vi "GOOP_LVClass_Global_OnCommand.vi"(10 "Command ID":string, 11 "Object":u64) -> ()   [LabVIEW 2020]
doc: "NI Confidential \n\n/**\n@brief This VI is called by the framework when the user selects a menu item on this item in the tree.\n\n@author Joel Dixon\n\n@par Sample_Item_OnCommand.vi\n The VI should contain a switch statement on the CommandID parameter to select the appropriate command and take the desired action for the command. See the description of the CommandID parameter for more information. \n\n@param \"Command ID\" [in] \nThe tag of the command to be performed. Corresponds to the Menu Tag field in the Menu Items cluster passed to mxLvSetPopupMenu.vi.\n*/"
uses:
  <resource>/Framework/Providers/Open_GDS/ClassProviders/Provider_BaseClassInterface/ClassWriter_class/ClassWriter.lvclass
  <resource>/Framework/Providers/Open_GDS/SubVIs/GOOP_UMLEditor_CallMainAction.ctl
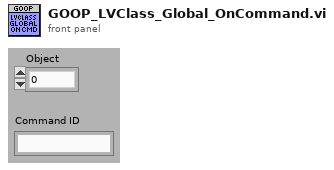
[diagram p1: front panel]
types:
  T1 = enum32{"None", "Stop", "Question", "Exclamation", "Information"}
  T2 = typedef "GOOP_UMLEditor_CallMainAction.ctl" = enum16{"OpenUmlEditor", "ReverseEngineering:WholeProject", "ReverseEngineering:OneClass", "ReverseEngineering:OneVI", "ShowInStateDiagram:OneVI", "OpenUMLFile"}
  T3 = enum32{"Bad", "Idle", "Run top level", "Running"}
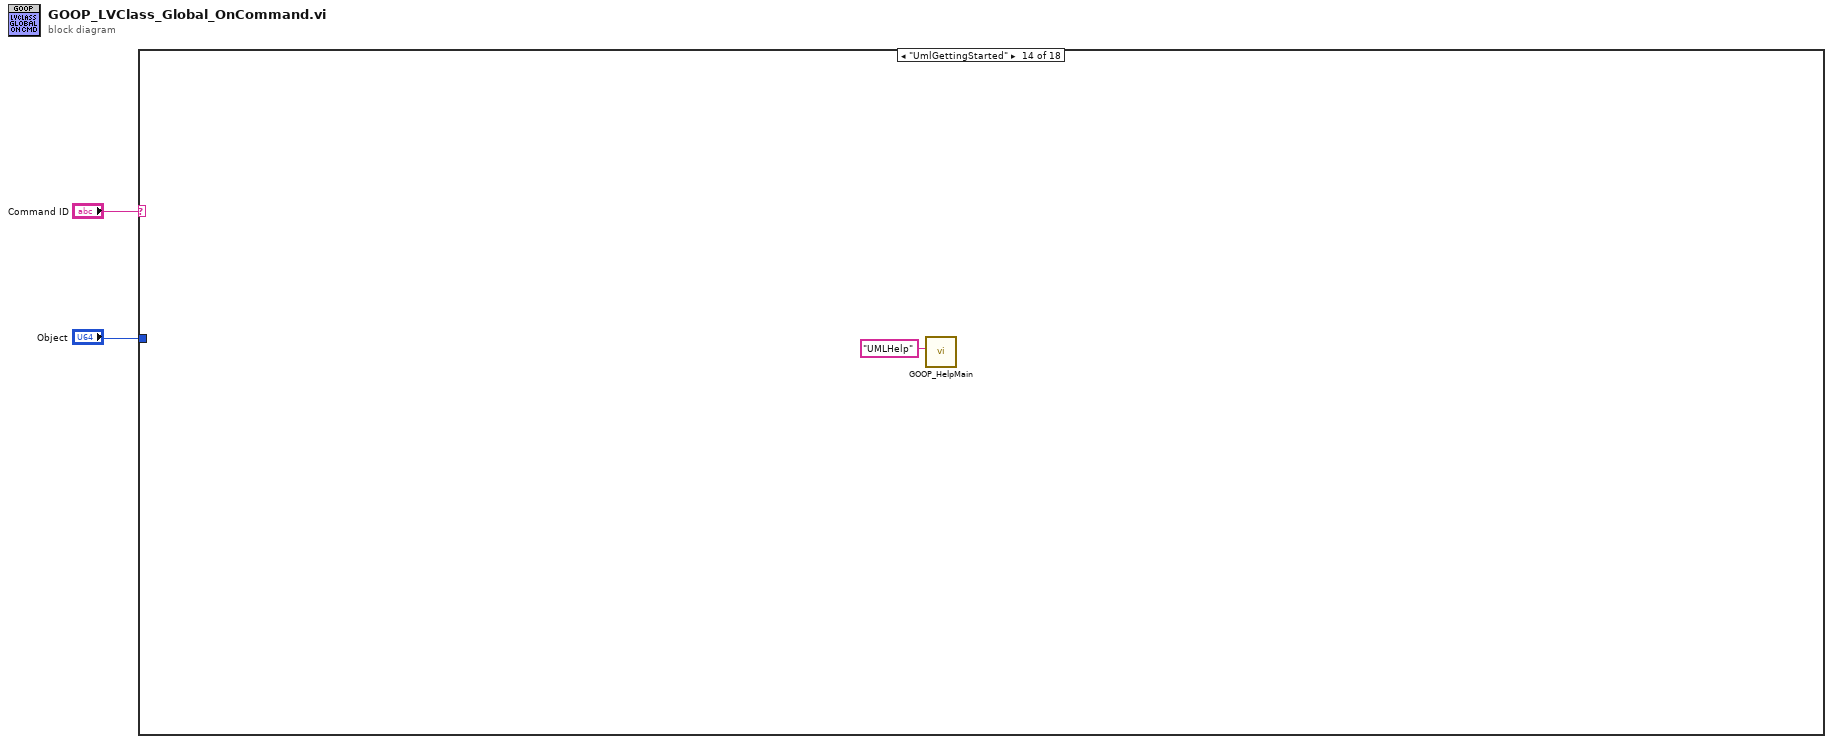
[diagram p0: block diagram]
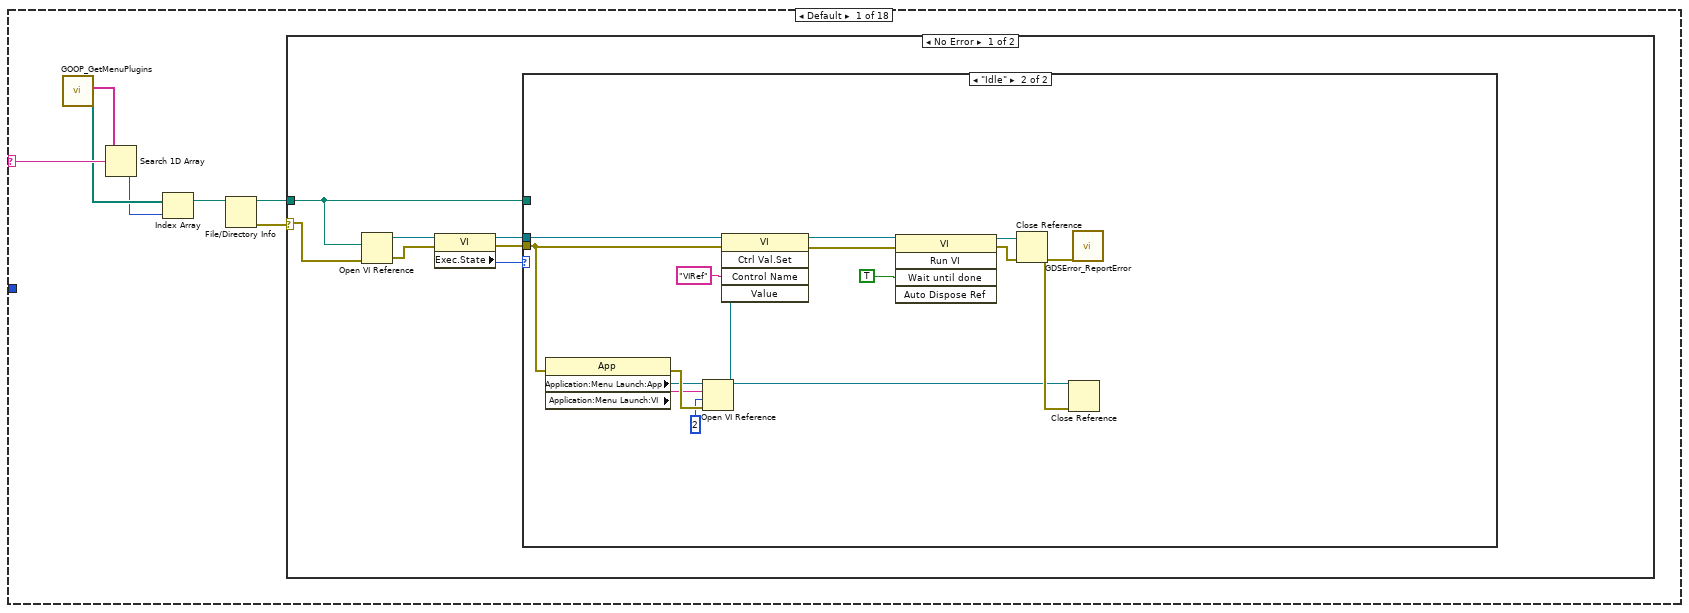
[diagram p2: hidden frame]
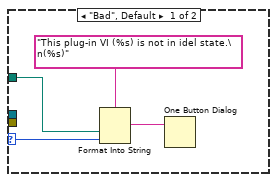
[diagram p3: hidden frame]
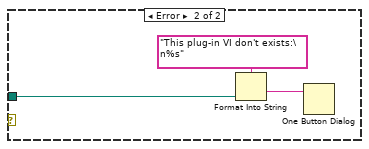
[diagram p4: hidden frame]
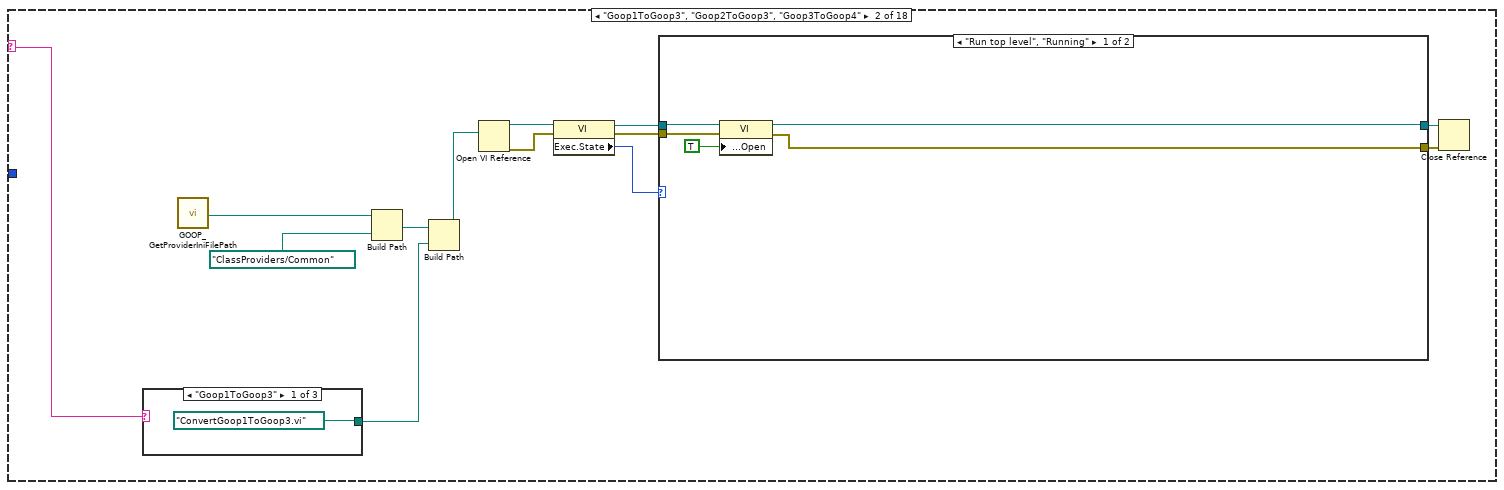
[diagram p5: hidden frame]
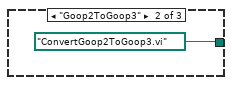
[diagram p6: hidden frame]
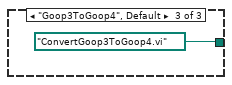
[diagram p7: hidden frame]
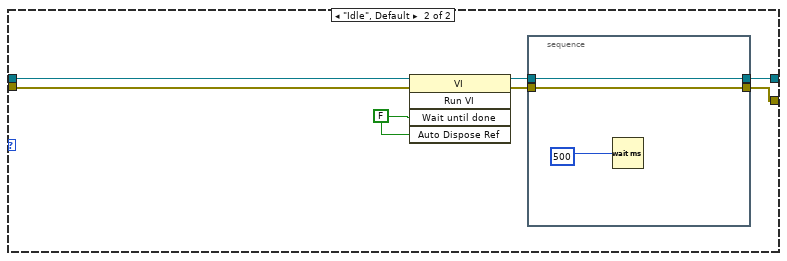
[diagram p8: hidden frame]
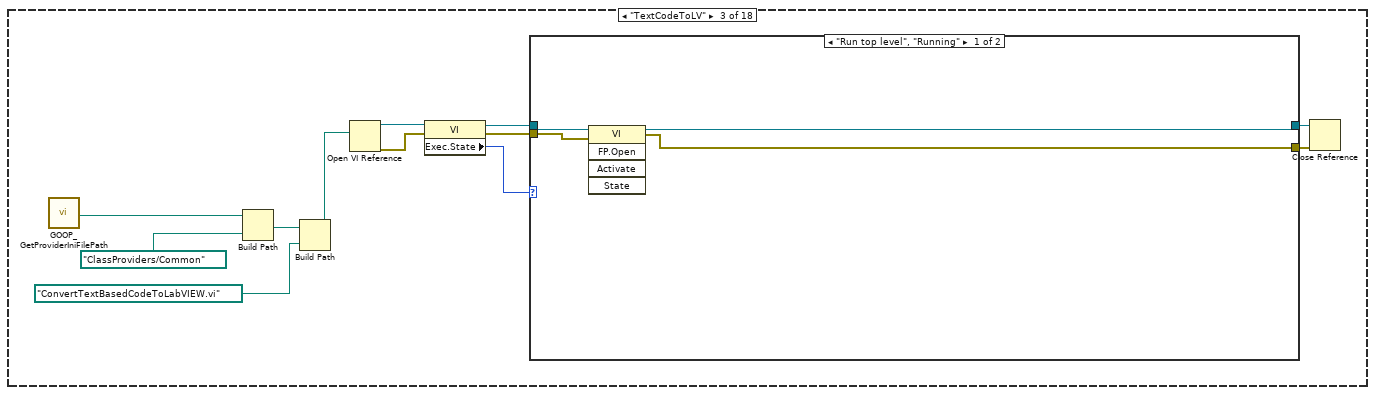
[diagram p9: hidden frame]
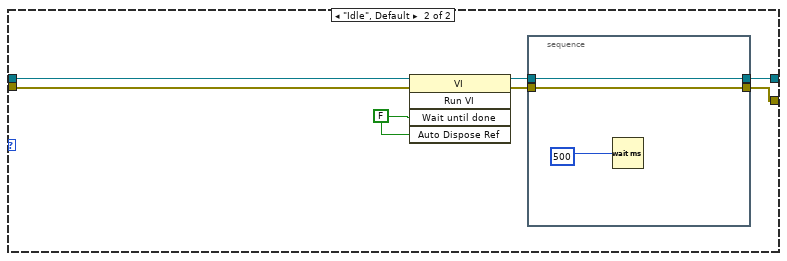
[diagram p10: hidden frame]
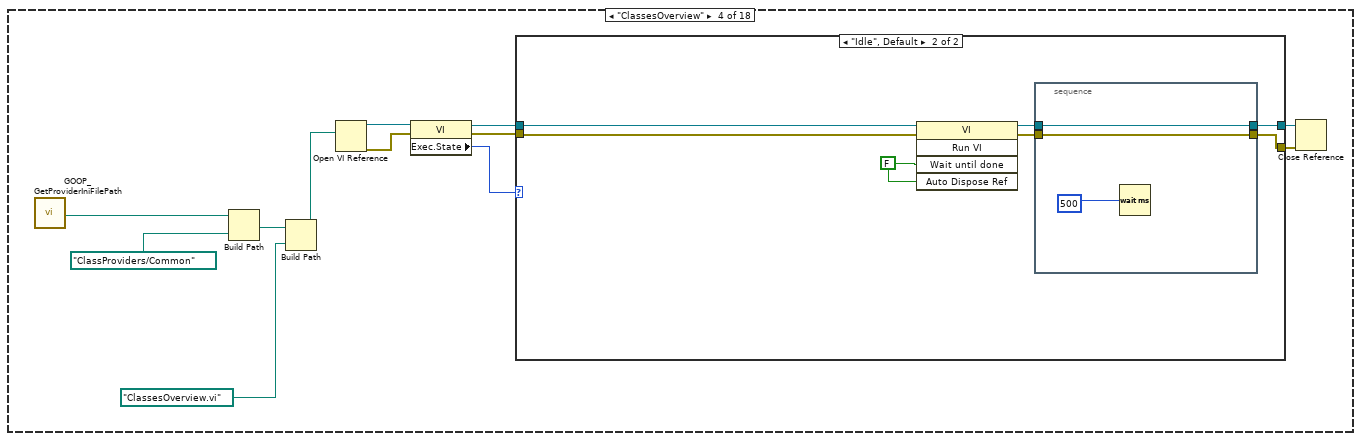
[diagram p11: hidden frame]
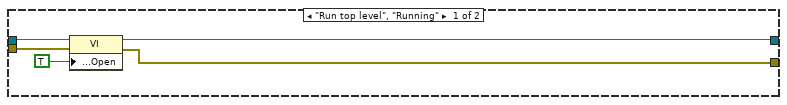
[diagram p12: hidden frame]
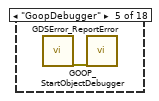
[diagram p13: hidden frame]
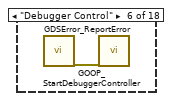
[diagram p14: hidden frame]
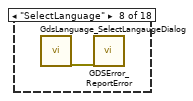
[diagram p16: hidden frame]
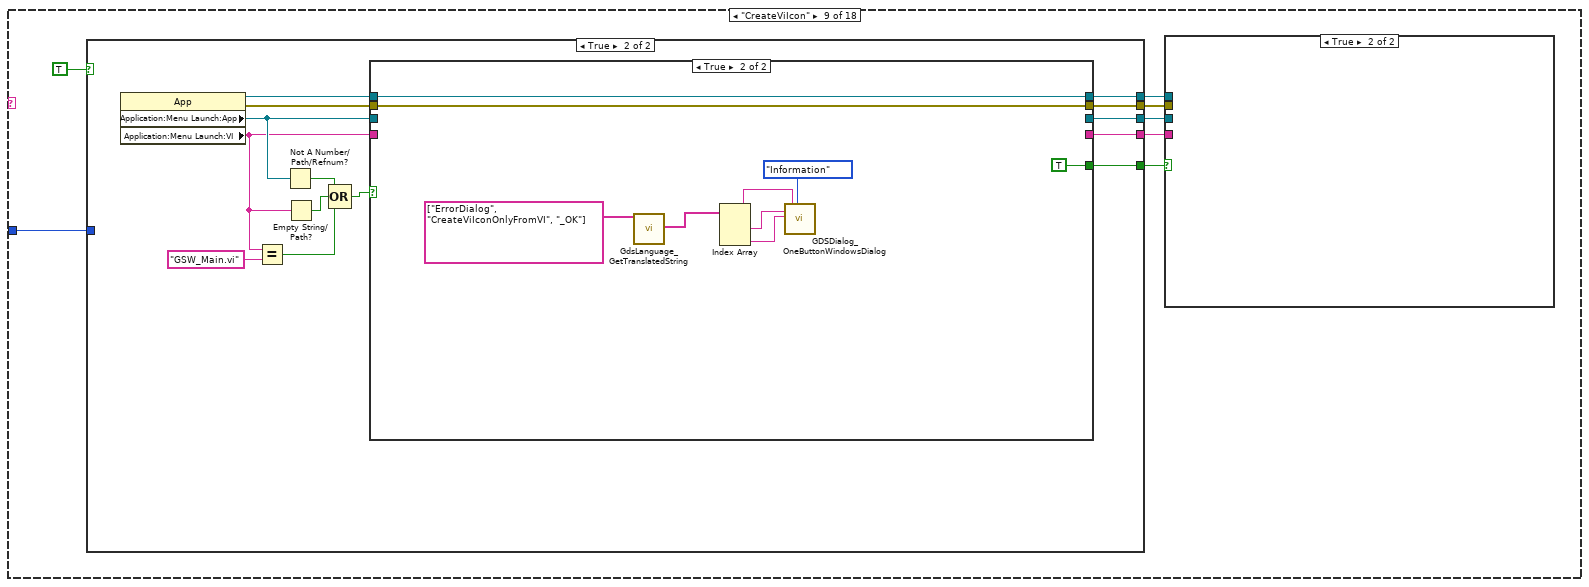
[diagram p17: hidden frame]
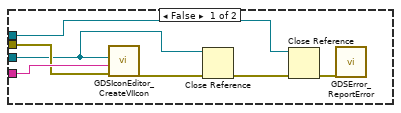
[diagram p18: hidden frame]
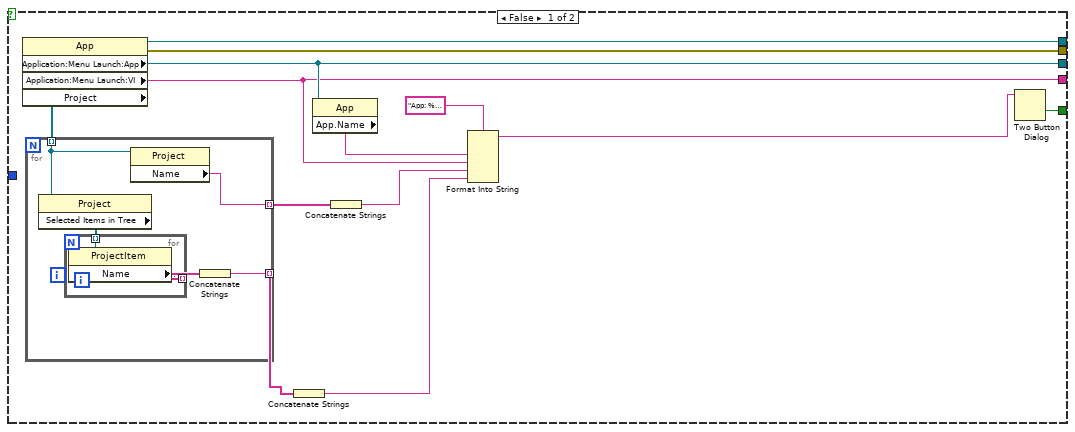
[diagram p19: hidden frame]
diagram:
  n1 = case shown="\"UmlGettingStarted\"" "Command ID" {
    selector: "Command ID" -> [w8 w40 _ _ _ _ _ _ _ _ _ w200 _ _ _ _ _ _]
    tunnel: "Object" -> [_ _ _ _ _ _ _ _ w125 _ _ w201 _ _ _ _ _ _]
    frame Default {
      n2 = call <resource>:"GOOP_GetMenuPlugins.vi"() -> ("MenuPluginsVIs"=w7:path[], "MenuPlugins(E.g. GOOP/My function)"=w9:string[])  [unwired: 10 in]
      n3 = Search 1D Array(1D array=w9, element=w8) -> (index of element=w6:i32)  [unwired: 1 in]
      n4 = Index Array(array=w7, index=w6) -> (element=w5:path)
      n5 = File/Directory Info(path=w5) -> (path out=w3:path, error out=w4:errorcluster)  [unwired: 1 in, 5 out]
      n6 = case shown="No Error" w4 {
        selector: w4 -> [w11 _]
        tunnel: w3 -> [w10 w35]
        frame No Error {
          n7 = Open VI Reference(vi path=w10, error in (no error)=w11) -> (vi reference=w13:refnum<vi>, error out=w12:errorcluster)  [unwired: 4 in]
          n8 = property class="VI"(reference=w13, error in=w12) -> (reference out=w15:refnum<vi>, error out=w14:errorcluster, "Exec.State"=w16:T3)
          n9 = case shown="\"Idle\"" w16 {
            selector: w16 -> [w17 _]
            tunnel: w10 -> [w18 _]
            tunnel: w15 -> [_ w31]
            tunnel: w14 -> [_ w23]
            frame "Bad", Default {
              n10 = Format Into String(format string="This plug-in VI (%s) is not in idel state.\n(%s)" ("message"), w18, w17) -> (resulting string=w20:string)  [unwired: 2 in, 1 out]
              n11 = One Button Dialog(message=w20) -> ()  [unwired: 1 in, 1 out]
            }
            frame "Idle" {
              n12 = property class="App"(error in=w23) -> (error out=w27:errorcluster, "Application:Menu Launch:App"=w25:refnum<vi>, "Application:Menu Launch:VI"=w26:string)  [unwired: 1 in, 1 out]
              n13 = Open VI Reference(application reference (local)=w25, vi path=w26, options=2, error in (no error)=w27) -> (vi reference=w21:refnum<vi>)  [unwired: 2 in, 1 out]
              n14 = invoke class="VI" method="Ctrl Val.Set"(reference=w31, error in=w23, "Control Name"="VIRef", "Value"=w21) -> (reference out=w30:refnum<vi>, error out=w29:errorcluster)  [unwired: 1 in, 3 out]
              n15 = invoke class="VI" method="Run VI"(reference=w30, error in=w29, "Wait until done"=TRUE ("Wait Until Done")) -> (reference out=w33:refnum<vi>, error out=w32:errorcluster)  [unwired: 2 in, 3 out]
              n16 = Close Reference(reference=w33, error in (no error)=w32) -> (error out=w22:errorcluster)
              n17 = Close Reference(reference=w21, error in (no error)=w22) -> ()  [unwired: 1 out]
              n18 = call <resource>:"GDSError_ReportError.vi"("error in (no error)"=w22) -> ()  [unwired: 18 in, 1 out]
            }
          }
        }
        frame Error {
          n19 = Format Into String(format string="This plug-in VI don't exists:\n%s" ("message"), w35) -> (resulting string=w37:string)  [unwired: 2 in, 1 out]
          n20 = One Button Dialog(message=w37) -> ()  [unwired: 1 in, 1 out]
        }
      }
    }
    frame "Goop1ToGoop3", "Goop2ToGoop3", "Goop3ToGoop4" {
      n21 = case shown="\"Goop1ToGoop3\"" w40 {
        tunnel: [path "ConvertGoop1ToGoop3.vi" ("base path") path "ConvertGoop2ToGoop3.vi" ("base path") path "ConvertGoop3ToGoop4.vi" ("base path")] -> w39
        frame "Goop1ToGoop3" {
        }
        frame "Goop2ToGoop3" {
        }
        frame "Goop3ToGoop4", Default {
        }
      }
      n22 = call <resource>:"GOOP_GetProviderIniFilePath.vi"() -> ("ProviderMainFolder"=w43:path)  [unwired: 10 in, 1 out]
      n23 = Build Path(base path=w43, name or relative path=path "ClassProviders/Common" ("base path")) -> (appended path=w42:path)
      n24 = Build Path(base path=w42, name or relative path=w39) -> (appended path=w41:path)
      n25 = Open VI Reference(vi path=w41) -> (vi reference=w47:refnum<vi>, error out=w48:errorcluster)  [unwired: 5 in]
      n26 = property class="VI"(reference=w47, error in=w48) -> (reference out=w45:refnum<vi>, error out=w46:errorcluster, "Exec.State"=w44:T3)
      n27 = case shown="\"Run top level\", \"Running\"" w44 {
        tunnel: [w54 w65] -> w50
        tunnel: [w55 w64] -> w49
        tunnel: w46 -> [w57 w59]
        tunnel: w45 -> [w58 w60]
        frame "Run top level", "Running" {
          n28 = property class="VI"(reference=w58, error in=w57, "Front Panel.Open"=TRUE ("Front Panel Window:Open")) -> (reference out=w55:refnum<vi>, error out=w54:errorcluster)
        }
        frame "Idle", Default {
          w61 = FALSE ("Wait Until Done")
          n29 = invoke class="VI" method="Run VI"(reference=w60, error in=w59, "Wait until done"=w61, "Auto Dispose Ref"=w61) -> (reference out=w63:refnum<vi>, error out=w62:errorcluster)  [unwired: 1 in, 3 out]
          n30 = stacked-sequence {
            tunnel: w62 -> [w67]
            tunnel: w63 -> [w68]
            tunnel: [w68] -> w64
            tunnel: [w67] -> w65
            frame #0 {
              n31 = Wait (ms)(milliseconds to wait=500) -> ()  [unwired: 1 out]
            }
          }
        }
      }
      n32 = Close Reference(reference=w49, error in (no error)=w50) -> ()  [unwired: 1 out]
    }
    frame "TextCodeToLV" {
      n33 = call <resource>:"GOOP_GetProviderIniFilePath.vi"() -> ("ProviderMainFolder"=w73:path)  [unwired: 10 in, 1 out]
      n34 = Build Path(base path=w73, name or relative path=path "ClassProviders/Common" ("base path")) -> (appended path=w72:path)
      n35 = Build Path(base path=w72, name or relative path=path "ConvertTextBasedCodeToLabVIEW.vi" ("base path")) -> (appended path=w71:path)
      n36 = Open VI Reference(vi path=w71) -> (vi reference=w77:refnum<vi>, error out=w78:errorcluster)  [unwired: 5 in]
      n37 = property class="VI"(reference=w77, error in=w78) -> (reference out=w75:refnum<vi>, error out=w76:errorcluster, "Exec.State"=w74:T3)
      n38 = case shown="\"Run top level\", \"Running\"" w74 {
        tunnel: [w81 w91] -> w80
        tunnel: [w82 w90] -> w79
        tunnel: w76 -> [w83 w85]
        tunnel: w75 -> [w84 w86]
        frame "Run top level", "Running" {
          n39 = invoke class="VI" method="FP.Open"(reference=w84, error in=w83) -> (reference out=w82:refnum<vi>, error out=w81:errorcluster)  [unwired: 3 in, 3 out]
        }
        frame "Idle", Default {
          w87 = FALSE ("Wait Until Done")
          n40 = invoke class="VI" method="Run VI"(reference=w86, error in=w85, "Wait until done"=w87, "Auto Dispose Ref"=w87) -> (reference out=w89:refnum<vi>, error out=w88:errorcluster)  [unwired: 1 in, 3 out]
          n41 = stacked-sequence {
            tunnel: w88 -> [w93]
            tunnel: w89 -> [w94]
            tunnel: [w94] -> w90
            tunnel: [w93] -> w91
            frame #0 {
              n42 = Wait (ms)(milliseconds to wait=500) -> ()  [unwired: 1 out]
            }
          }
        }
      }
      n43 = Close Reference(reference=w79, error in (no error)=w80) -> ()  [unwired: 1 out]
    }
    frame "ClassesOverview" {
      n44 = call <resource>:"GOOP_GetProviderIniFilePath.vi"() -> ("ProviderMainFolder"=w100:path)  [unwired: 10 in, 1 out]
      n45 = Build Path(base path=w100, name or relative path=path "ClassProviders/Common" ("base path")) -> (appended path=w99:path)
      n46 = Build Path(base path=w99, name or relative path=path "ClassesOverview.vi" ("base path")) -> (appended path=w96:path)
      n47 = Open VI Reference(vi path=w96) -> (vi reference=w103:refnum<vi>, error out=w104:errorcluster)  [unwired: 5 in]
      n48 = property class="VI"(reference=w103, error in=w104) -> (reference out=w101:refnum<vi>, error out=w102:errorcluster, "Exec.State"=w97:T3)
      n49 = case shown="\"Idle\", Default" w97 {
        tunnel: [w107 w118] -> w106
        tunnel: [w108 w117] -> w105
        tunnel: w102 -> [w110 w112]
        tunnel: w101 -> [w111 w113]
        frame "Run top level", "Running" {
          n50 = property class="VI"(reference=w111, error in=w110, "Front Panel.Open"=TRUE ("Front Panel Window:Open")) -> (reference out=w108:refnum<vi>, error out=w107:errorcluster)
        }
        frame "Idle", Default {
          w114 = FALSE ("Wait Until Done")
          n51 = invoke class="VI" method="Run VI"(reference=w113, error in=w112, "Wait until done"=w114, "Auto Dispose Ref"=w114) -> (reference out=w116:refnum<vi>, error out=w115:errorcluster)  [unwired: 1 in, 3 out]
          n52 = stacked-sequence {
            tunnel: w115 -> [w120]
            tunnel: w116 -> [w121]
            tunnel: [w121] -> w117
            tunnel: [w120] -> w118
            frame #0 {
              n53 = Wait (ms)(milliseconds to wait=500) -> ()  [unwired: 1 out]
            }
          }
        }
      }
      n54 = Close Reference(reference=w105, error in (no error)=w106) -> ()  [unwired: 1 out]
    }
    frame "GoopDebugger" {
      n55 = call <resource>:"GOOP_StartObjectDebugger.vi"() -> ("error out"=w122:errorcluster)  [unwired: 19 in]
      n56 = call <resource>:"GDSError_ReportError.vi"("error in (no error)"=w122) -> ()  [unwired: 18 in, 1 out]
    }
    frame "Debugger Control" {
      n57 = call <resource>:"GOOP_StartDebuggerController.vi"() -> ("error out"=w123:errorcluster)  [unwired: 19 in]
      n58 = call <resource>:"GDSError_ReportError.vi"("error in (no error)"=w123) -> ()  [unwired: 18 in, 1 out]
    }
    frame "OpenGDebugger" {
    }
    frame "SelectLanguage" {
      n59 = call <resource>:"GdsLanguage_SelectLangaugeDialog.vi"() -> ("error out"=w124:errorcluster)  [unwired: 18 in, 1 out]
      n60 = call <resource>:"GDSError_ReportError.vi"("error in (no error)"=w124) -> ()  [unwired: 18 in, 1 out]
    }
    frame "CreateViIcon" {
      n61 = case shown="True" TRUE {
        tunnel: [w149 w167] -> w131
        tunnel: [w145 w166] -> w130
        tunnel: [w150 w165] -> w128
        tunnel: [w151 w163] -> w127
        tunnel: [w148 w164] -> w126
        tunnel: w125 -> [_ _]
        frame False {
          n62 = property class="App"() -> (reference out=w150:refnum<vi>, error out=w151:errorcluster, "Application:Menu Launch:App"=w149:refnum<vi>, "Application:Menu Launch:VI"=w145:string, "Project"=w143:refnum<vi>[])  [unwired: 2 in]
          n63 = for {
            tunnel: w143 -> [w153] mode=indexing
            tunnel: [w154] -> w142 mode=indexing
            tunnel: [w152] -> w140 mode=indexing
            n64 = property class="Project"(reference=w153) -> ("Selected Items in Tree"=w156:refnum<vi>[])  [unwired: 1 in, 2 out]
            n65 = for {
              tunnel: w156 -> [w158] mode=indexing
              tunnel: [w157] -> w155 mode=indexing
              n66 = property class="ProjectItem"(reference=w158) -> ("Name"=w157:string)  [unwired: 1 in, 2 out]
            }
            n67 = property class="Project"(reference=w153) -> ("Name"=w152:string)  [unwired: 1 in, 2 out]
            n68 = Concatenate Strings(w155) -> (w154:string)
          }
          n69 = Concatenate Strings(w142) -> (w141:string)
          n70 = property class="App"(reference=w149) -> ("App.Name"=w146:string)  [unwired: 1 in, 2 out]
          n71 = Concatenate Strings(w140) -> (w139:string)
          n72 = Format Into String(format string="App: %s\nVI: %s\nProjectType:%s\nProjectItemName: %s", w146, w145, w139, w141) -> (resulting string=w144:string)  [unwired: 2 in, 1 out]
          n73 = Two Button Dialog(message=w144) -> (T button?=w148:bool)  [unwired: 2 in]
        }
        frame True {
          n74 = property class="App"() -> (reference out=w169:refnum<vi>, error out=w170:errorcluster, "Application:Menu Launch:App"=w168:refnum<vi>, "Application:Menu Launch:VI"=w161:string)  [unwired: 2 in]
          n75 = Equal?(x=w161, y="GSW_Main.vi") -> (x = y?=w159:bool)
          n76 = Not A Number/Path/Refnum?(number/path/refnum=w168) -> (NaN/Path/Refnum?=w172:bool)
          n77 = Empty String/Path?(string/path=w161) -> (empty?=w162:bool)
          n78 = Compound Arithmetic op=OR(w172, w162, w159) -> (w171:bool)
          n79 = case shown="True" w171 {
            tunnel: w170 -> [w173 w184]
            tunnel: w169 -> [w174 w185]
            tunnel: w168 -> [w176 _]
            tunnel: w161 -> [w175 _]
            tunnel: [w176 _] -> w167
            tunnel: [w175 _] -> w166
            tunnel: [w174 w185] -> w165
            tunnel: [_ TRUE] -> w164
            tunnel: [w173 w184] -> w163
            frame False {
            }
            frame True {
              n80 = call <resource>:"GdsLanguage_GetTranslatedString.vi"("StringID(s)"=string[] ["ErrorDialog", "CreateViIconOnlyFromVI", "_OK"]) -> ("StringsOut"=w180:string[])  [unwired: 15 in, 3 out]
              n81 = Index Array(array=w180) -> (element #1=w179:string, element #2=w178:string, element #3=w177:string)  [unwired: 3 in]
              n82 = call <resource>:"GDSDialog_OneButtonWindowsDialog.vi"("UserText"=w178, "ButtonName"=w177, "DialogTitle"=w179, "Icon"=T1."Information") -> ()  [unwired: 13 in, 3 out]
            }
          }
        }
      }
      n83 = case shown="True" w126 {
        tunnel: w131 -> [w133 _]
        tunnel: w130 -> [w138 _]
        tunnel: w128 -> [w137 _]
        tunnel: w127 -> [w136 _]
        frame False {
          n84 = call <resource>:"GDSIconEditor_CreateVIIcon.vi"("error in (no error)"=w136, "Application:Menu Launch:VI"=w138, "Application:Menu Launch:App"=w133) -> ("error out"=w134:errorcluster)  [unwired: 8 in]
          n85 = Close Reference(reference=w133, error in (no error)=w134) -> (error out=w135:errorcluster)
          n86 = Close Reference(reference=w137, error in (no error)=w135) -> (error out=w132:errorcluster)
          n87 = call <resource>:"GDSError_ReportError.vi"("error in (no error)"=w132) -> ()  [unwired: 18 in, 1 out]
        }
        frame True {
        }
      }
    }
    frame "GoopOptions" {
      n88 = call <resource>:"ClassProvidor_GoopOptionsDialog.vi"() -> ("error out"=w186:errorcluster)  [unwired: 11 in]
      n89 = call <resource>:"GDSError_ReportError.vi"("error in (no error)"=w186) -> ()  [unwired: 18 in, 1 out]
    }
    frame "ActorOptions" {
      n90 = call <resource>:"AF_Configuration.vi"() -> ("Error Out"=w187:errorcluster)  [unwired: 19 in]
      n91 = call <resource>:"GDSError_ReportError.vi"("error in (no error)"=w187) -> ()  [unwired: 18 in, 1 out]
    }
    frame "OpenUmlModeller", "ViewViInStateDiagram" {
      n92 = call <resource>:"mxLvGetItemRef.vi"("Item"=w201) -> ("Item Refnum"=w221:refnum<vi>, "error out"=w212:errorcluster)  [unwired: 1 in, 1 out]
      n93 = property class="ProjectItem"(reference=w221, error in=w212) -> (reference out=w216:refnum<vi>, error out=w213:errorcluster, "Project"=w220:refnum<vi>, "Type String"=w214:string, "Target"=w190:refnum<vi>)
      n94 = case shown="\"LvClass\"" w214 {
        tunnel: w216 -> [w233 w239 w245]
        tunnel: [w233 w235 w241] -> w215
        tunnel: [_ w234 w240] -> w193
        frame Default {
        }
        frame "LvClass" {
          w238 = refnum<vi> refnum  # LVClassLibrary
          n95 = To More Specific Class(target class=w238, reference=w239) -> (specific class reference=w237:refnum<vi>, error out=w236:errorcluster)  [unwired: 1 in]
          n96 = property class="LVClassLibrary"(reference=w237, error in=w236) -> (reference out=w235:refnum<vi>, "Path"=w234:path)  [unwired: 1 out]
        }
        frame "VI" {
          w244 = refnum<vi> refnum  # ProjectItem
          n97 = To More Specific Class(target class=w244, reference=w245) -> (specific class reference=w243:refnum<vi>, error out=w242:errorcluster)  [unwired: 1 in]
          n98 = property class="ProjectItem"(reference=w243, error in=w242) -> (reference out=w241:refnum<vi>, "Path"=w240:path)  [unwired: 1 out]
        }
      }
      n99 = property class="TargetItem"(reference=w190) -> (reference out=w189:refnum<vi>, "Name"=w188:string)  [unwired: 1 in, 1 out]
      n100 = property class="Project"(reference=w220, error in=w213) -> (reference out=w218:refnum<vi>, error out=w219:errorcluster, "Name"=w194:string)
      n101 = Close Reference(reference=w218, error in (no error)=w219) -> (error out=w217:errorcluster)
      n102 = Close Reference(reference=w189) -> ()  [unwired: 1 in, 1 out]
      n103 = Equal?(x=w200, y="ViewViInStateDiagram") -> (x = y?=w198:bool)
      n104 = Close Reference(reference=w215, error in (no error)=w217) -> ()  [unwired: 1 out]
      n105 = Select(t=GOOP_UMLEditor_CallMainAction."ShowInStateDiagram:OneVI" ("Enum"), s=w198, f=GOOP_UMLEditor_CallMainAction."OpenUmlEditor" ("Enum")) -> (s? t:f=w195:T2)
      n106 = call-dynamic "Init.vi"("ClassWriter in"=refnum<class "ClassWriter.lvclass"> refnum) -> ("ClassWriter out"=w204:refnum<class "ClassWriter.lvclass">, "error out"=w208:errorcluster)  [unwired: 17 in]
      n107 = case shown="\"ShowInStateDiagram:OneVI\"" w195 {
        tunnel: w194 -> [w223 _]
        tunnel: w193 -> [w222 _]
        tunnel: [w223 w227] -> w192
        tunnel: [w222 w226] -> w191
        frame Default {
        }
        frame "ShowInStateDiagram:OneVI" {
          n108 = property class="App"() -> ("Application:Menu Launch:App"=w231:refnum<vi>, "Application:Menu Launch:VI"=w232:string)  [unwired: 2 in, 2 out]
          n109 = Open VI Reference(application reference (local)=w231, vi path=w232, options=2) -> (vi reference=w229:refnum<vi>, error out=w228:errorcluster)  [unwired: 3 in]
          n110 = property class="VI"(reference=w229, error in=w228) -> (reference out=w224:refnum<vi>, error out=w225:errorcluster, "Name"=w227:string, "Path"=w226:path)
          n111 = Close Reference(reference=w224, error in (no error)=w225) -> ()  [unwired: 1 out]
        }
      }
      n112 = call <resource>:"GdsLanguage_GetTranslatedString.vi"("StringID(s)"="OpenUmlModeller" ("Message(Exit)"), "error in (no error)"=w208) -> ("FirstStringOut"=w211:string, "error out"=w210:errorcluster)  [unwired: 14 in, 2 out]
      n113 = call-dynamic "ProgressWindow.vi"("ClassWriter in"=w204, "Message(Exit)"=w211, "error in (no error)"=w210) -> ("ClassWriter out"=w205:refnum<class "ClassWriter.lvclass">, "error out"=w207:errorcluster)  [unwired: 15 in]
      n114 = call <resource>:"GOOP_UMLEditor_CallMain.vi"("Enum"=w195, "Project"=w192, "Class/VI-Path"=w191, "Target"=w188, "error in (no error)"=w207) -> ("error out"=w206:errorcluster)  [unwired: 14 in]
      n115 = call-dynamic "Destroy.vi"("ClassWriter.lvclass"=w205, "error in (no error)"=w206) -> ("error out"=w203:errorcluster)  [unwired: 17 in]
      n116 = call <resource>:"GDSError_ReportError.vi"("error in (no error)"=w203) -> ()  [unwired: 18 in, 1 out]
    }
    frame "UMLOpen" {
      n117 = disable-structure shown="Enabled" {
        frame Enabled {
          n118 = call-dynamic "Init.vi"("ClassWriter in"=refnum<class "ClassWriter.lvclass"> refnum) -> ("ClassWriter out"=w249:refnum<class "ClassWriter.lvclass">, "error out"=w253:errorcluster)  [unwired: 17 in]
          n119 = call <resource>:"GdsLanguage_GetTranslatedString.vi"("StringID(s)"="OpenUmlModeller" ("Message(Exit)"), "error in (no error)"=w253) -> ("FirstStringOut"=w256:string, "error out"=w255:errorcluster)  [unwired: 14 in, 2 out]
          n120 = call-dynamic "ProgressWindow.vi"("ClassWriter in"=w249, "Message(Exit)"=w256, "error in (no error)"=w255) -> ("ClassWriter out"=w250:refnum<class "ClassWriter.lvclass">, "error out"=w252:errorcluster)  [unwired: 15 in]
          n121 = call <resource>:"GOOP_UMLEditor_CallMain.vi"("Enum"=GOOP_UMLEditor_CallMainAction."OpenUmlEditor", "error in (no error)"=w252) -> ("error out"=w251:errorcluster)  [unwired: 17 in]
          n122 = call-dynamic "Destroy.vi"("ClassWriter.lvclass"=w250, "error in (no error)"=w251) -> ("error out"=w248:errorcluster)  [unwired: 17 in]
          n123 = call <resource>:"GDSError_ReportError.vi"("error in (no error)"=w248) -> ()  [unwired: 18 in, 1 out]
        }
        frame Disabled {
        }
      }
    }
    frame "UmlGettingStarted" {
      n124 = call <resource>:"GOOP_HelpMain.vi"("File"="UMLHelp") -> ()  [unwired: 11 in]
    }
    frame "ActivateProduct" {
    }
    frame "ProductInfo" {
      n125 = call <resource>:"OpenGDSLicense_ProductInfo.vi"() -> ("error out"=w258:errorcluster)  [unwired: 19 in]
      n126 = call <resource>:"GDSError_ReportError.vi"("error in (no error)"=w258) -> ()  [unwired: 18 in, 1 out]
    }
    frame "GettingStarted" {
      n127 = call <resource>:"GOOP_HelpMain.vi"("File"="GettingStarted") -> ()  [unwired: 11 in]
    }
    frame "MenuHelp" {
      n128 = call <resource>:"GOOP_HelpMain.vi"("File"="MainHelp") -> ()  [unwired: 11 in]
    }
  }
